vi "Turbine Flow.vi"(0 "Structure Area (m²)":i32, 1 "Energy Needed (FE)":ext, 5 "Inner Area (m²)":i32, 7 "Rotor Height (m)":i32, 9 "Blades":i32, 11 "Stored Gas (mB/t)":i64, 12 "Coils":i32, 13 "Vents":i32) -> (3 "Energy Production (FE/t)":ext, 4 "Flow (mB/t)":i64, 6 "Vents Limiting":bool, 8 "Dispersers Limiting":bool, 10 "Blades Limiting":bool, 14 "Rotation":dbl, 15 "Coils Limiting":bool)   [LabVIEW 2023]
uses:
  cdebc2e5-f1fa-de40-91d8-d9d568490e02.vi
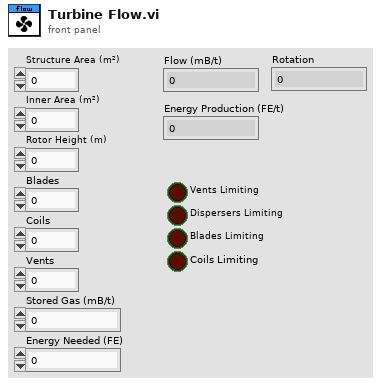
[diagram p1: front panel]
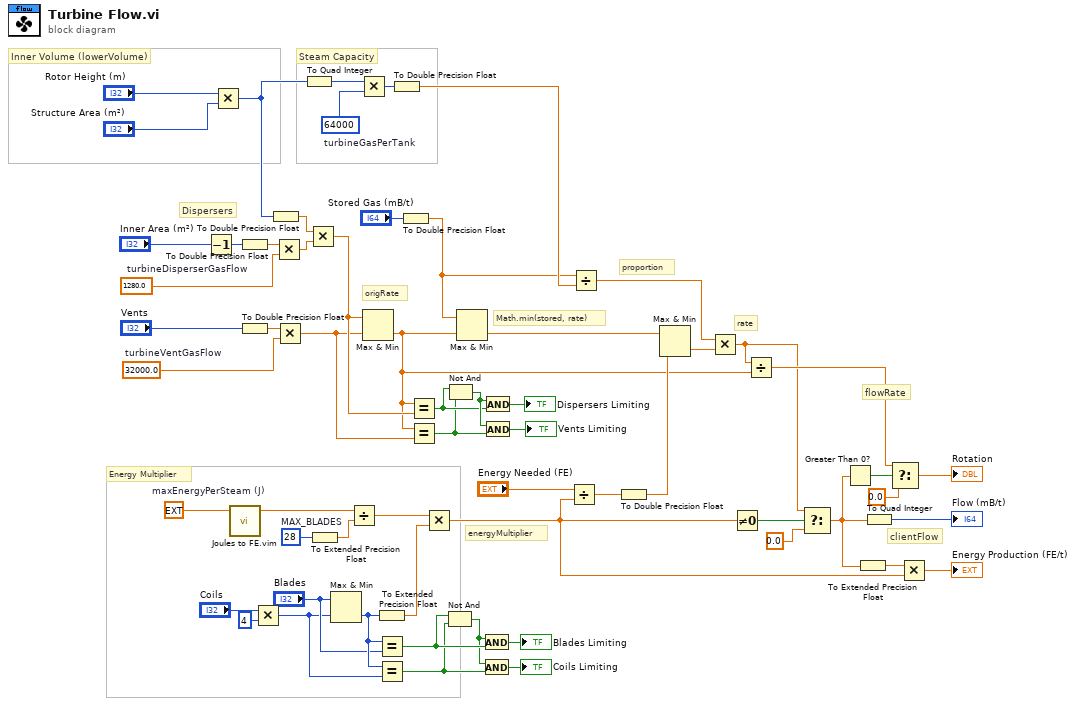
[diagram p0: block diagram]
diagram:
  w48 = i64 64000  # turbineGasPerTank
  w54 = 28  # MAX_BLADES
  w18 = ext 10.0  # maxEnergyPerSteam (J)
  w57 = 32000.0  # turbineVentGasFlow
  w59 = 1280.0  # turbineDisperserGasFlow
  # "Math.min(stored, rate)"
  # "flowRate"
  # "clientFlow"
  # "energyMultiplier"
  # "rate"
  # "origRate"
  # "Dispersers"
  # "proportion"
  # "Steam Capacity"
  # "Energy Multiplier"
  # "Inner Volume (lowerVolume)"
  n1 = Decrement(x="Inner Area (m²)") -> (x-1=w12:i32)
  n2 = Multiply(x="Rotor Height (m)", y="Structure Area (m²)") -> (x*y=w23:i32)
  n3 = call "Joules to FE.vim"("J"=w18) -> ("FE"=w22:ext)  [unwired: 4 in]
  n4 = To Double Precision Float(number=w12) -> (double precision float=w11:dbl)
  n5 = To Double Precision Float(number="Vents") -> (double precision float=w20:dbl)
  n6 = Multiply(x="Coils", y=4) -> (x*y=w35:i32)
  n7 = To Double Precision Float(number=w23) -> (double precision float=w10:dbl)
  n8 = Multiply(x=w11, y=w59) -> (x*y=w56:dbl)
  n9 = Multiply(x=w20, y=w57) -> (x*y=w38:dbl)
  n10 = To Quad Integer(1:w23) -> (0:w21:i64)
  n11 = Multiply(x=w10, y=w56) -> (x*y=w39:dbl)
  n12 = To Extended Precision Float(1:w54) -> (0:w55:ext)
  n13 = Max & Min(x="Blades", y=w35) -> (min(x,y)=w37:i32)  [unwired: 1 out]
  n14 = Divide(x=w22, y=w55) -> (x/y=w53:ext)
  n15 = Multiply(x=w21, y=w48) -> (x*y=w45:i64)
  n16 = Max & Min(x=w39, y=w38) -> (min(x,y)=w13:dbl)  [unwired: 1 out]
  n17 = To Extended Precision Float(1:w37) -> (0:w50:ext)
  n18 = Equal?(x=w37, y="Blades") -> (x = y?=w34:bool)
  n19 = Equal?(x=w37, y=w35) -> (x = y?=w31:bool)
  n20 = To Double Precision Float(number=w45) -> (double precision float=w44:dbl)
  n21 = To Double Precision Float(number="Stored Gas (mB/t)") -> (double precision float=w19:dbl)
  n22 = Equal?(x=w13, y=w39) -> (x = y?=w28:bool)
  n23 = Equal?(x=w13, y=w38) -> (x = y?=w27:bool)
  n24 = Multiply(x=w53, y=w50) -> (x*y=w3:ext)
  n25 = Not And(1:w31, 2:w34) -> (0:w32:bool)
  n26 = Not And(1:w27, 2:w28) -> (0:w29:bool)
  n27 = Max & Min(x=w19, y=w13) -> (min(x,y)=w14:dbl)  [unwired: 1 out]
  n28 = And(x=w32, y=w34) -> (x .and. y?=→"Blades Limiting":bool)
  n29 = And(x=w32, y=w31) -> (x .and. y?=→"Coils Limiting":bool)
  n30 = And(x=w29, y=w28) -> (x .and. y?=→"Dispersers Limiting":bool)
  n31 = And(x=w29, y=w27) -> (x .and. y?=→"Vents Limiting":bool)
  n32 = Divide(x="Energy Needed (FE)", y=w3) -> (x/y=w41:ext)
  n33 = Divide(x=w19, y=w44) -> (x/y=w43:dbl)
  n34 = To Double Precision Float(number=w41) -> (double precision float=w17:dbl)
  n35 = Max & Min(x=w14, y=w17) -> (min(x,y)=w42:dbl)  [unwired: 1 out]
  n36 = Multiply(x=w43, y=w42) -> (x*y=w9:dbl)
  n37 = Not Equal To 0?(x=w3) -> (x != 0?=w49:bool)
  n38 = Divide(x=w9, y=w13) -> (x/y=w60:dbl)
  n39 = Select(t=w9, s=w49, f=0.0 ("Stored Gas (mB/t)")) -> (s? t:f=w4:dbl)
  n40 = Greater Than 0?(x=w4) -> (x > 0?=w16:bool)
  n41 = To Extended Precision Float(1:w4) -> (0:w2:ext)
  n42 = To Quad Integer(1:w4) -> (0:→"Flow (mB/t)":i64)
  n43 = Select(t=w60, s=w16, f=0.0) -> (s? t:f=→"Rotation":dbl)
  n44 = Multiply(x=w2, y=w3) -> (x*y=→"Energy Production (FE/t)":ext)
